vi "Setup UI.vi"(8 "error in (no error)":errorcluster, 10 "Set UI to input? (F)":bool, 11 "Wavelength in":refnum<class "Wavelength.lvclass">) -> (0 "error out":errorcluster, 3 "Wavelength out":refnum<class "Wavelength.lvclass">)   [LabVIEW 2012, in "Wavelength.lvclass"]
uses:
  Wavelength.lvclass
  Wavelength.lvclass/Wavelength.ctl
  Instruments/Spectrometer/Spectrometer Triax 550.lvclass
  Instruments/Spectrometer/JY-SPEX-TRIAX/JY-SPEX-TRIAX.lvlib
panel:
  in  "Set mirror (lateral)":bool
  in  "Go to first point":bool
  in  "Optimize":enum32{"Slits", "Step Size"}(radio)=enum."Step Size"
  out "Step size":dbl[unit] caption="Recommended step size\n(must enter above too)"
  in  "Lateral Exit":dbl[unit]
  in  "Axial Entrance":dbl[unit]
  # "Wavelength Scan Setup"
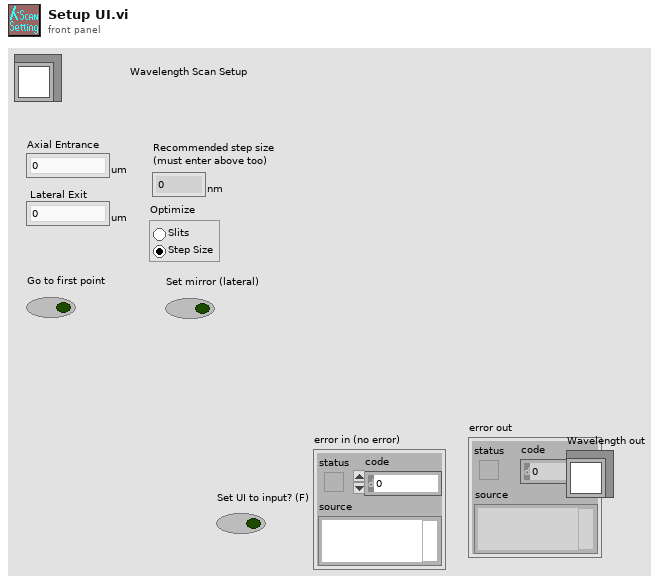
[diagram p1: front panel]
types:
  T1 = enum8{"Enabled", "Disabled", "Disabled and Grayed Out"}
  T2 = typedef "Scanner.lvclass/Range.ctl" = cluster{"xi":dbl, "xf":dbl, "dx":dbl, "Return to...?":bool, "Return to":dbl}
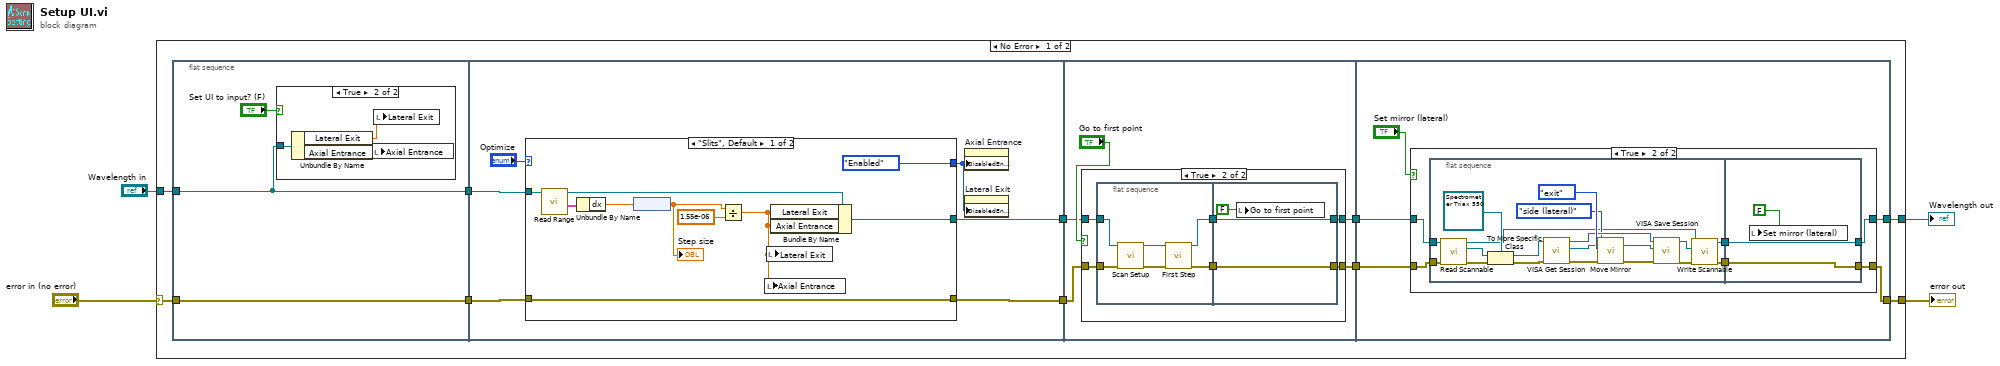
[diagram p0: block diagram]
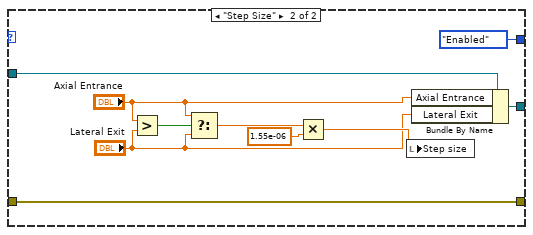
[diagram p3: hidden frame]
diagram:
  n1 = case shown="No Error" "error in (no error)" {
    selector: "error in (no error)" -> [w13 w104]
    tunnel: [w14 w104] -> w3
    tunnel: "Wavelength in" -> [w12 w105]
    tunnel: [w11 w105] -> w1
    frame No Error {
      n2 = flat-sequence {
        tunnel: w12 -> [w15]
        tunnel: w13 -> [w17]
        tunnel: [w17] -> w10
        tunnel: [w15] -> w9
        tunnel: w10 -> [w24]
        tunnel: w9 -> [w23]
        tunnel: [w25] -> w8
        tunnel: [w22] -> w7
        tunnel: w8 -> [w49]
        tunnel: w7 -> [w50]
        tunnel: [w48] -> w6
        tunnel: [w47] -> w5
        tunnel: [w73] -> w11
        tunnel: [w70] -> w14
        tunnel: w6 -> [w72]
        tunnel: w5 -> [w71]
        frame #0 {
          n3 = case shown="True" "Set UI to input? (F)" {
            tunnel: w15 -> [_ w20]
            frame False {
            }
            frame True {
              n4 = Unbundle By Name(w20) -> ("Lateral Exit"=w19:dbl[unit], "Axial Entrance"=w18:dbl[unit])
              n5 = local write "Axial Entrance"(w18) -> ()
              n6 = local write "Lateral Exit"(w19) -> ()
            }
          }
        }
        frame #1 {
          n7 = case shown="\"Slits\", Default" "Optimize" {
            tunnel: [w35 w42] -> w25
            tunnel: w24 -> [w35 w42]
            tunnel: w23 -> [w34 w43]
            tunnel: [w33 w40] -> w22
            tunnel: [T1."Enabled" ("Disabled") T1."Enabled" ("Disabled")] -> w21
            frame "Slits", Default {
              n8 = call-dynamic "Read Range.vi"("Scanner.lvclass in"=w34) -> ("Range"=w30:T2, "Scanner.lvclass out"=w31:refnum<class "Wavelength.lvclass">)  [unwired: 5 in, 4 out]
              n9 = Unbundle By Name(w30) -> ("dx"=w29:dbl)
              n10 = node(w29) -> (w28:dbl[unit])
              "Step size" <- w28
              n11 = Divide(x=w28, y=1.55e-06) -> (x/y=w32:dbl[unit])
              n12 = local write "Axial Entrance"(w32) -> ()
              n13 = local write "Lateral Exit"(w32) -> ()
              n14 = Bundle By Name(cluster=w31, "Lateral Exit"=w32, "Axial Entrance"=w32) -> (w33:refnum<class "Wavelength.lvclass">)
            }
            frame "Step Size" {
              n15 = Greater?(x="Axial Entrance", y="Lateral Exit") -> (0:w45:bool)
              n16 = Select(t="Axial Entrance", s=w45, f="Lateral Exit") -> (s? t:f=w44:dbl[unit])
              n17 = Multiply(x=w44, y=1.55e-06) -> (x*y=w41:dbl[unit])
              n18 = local write "Step size"(w41) -> ()
              n19 = Bundle By Name(cluster=w43, "Axial Entrance"="Axial Entrance", "Lateral Exit"="Lateral Exit") -> (w40:refnum<class "Wavelength.lvclass">)
            }
          }
          n20 = property on="Axial Entrance" class="DigNum (strict)"("DisabledEnum"=w21) -> ()  [unwired: 2 in, 2 out]
          n21 = property on="Lateral Exit" class="DigNum (strict)"("DisabledEnum"=w21) -> ()  [unwired: 2 in, 2 out]
        }
        frame #2 {
          n22 = case shown="True" "Go to first point" {
            tunnel: w50 -> [w53 w59]
            tunnel: w49 -> [w52 w58]
            tunnel: [w52 w57] -> w47
            tunnel: [w53 w56] -> w48
            frame False {
            }
            frame True {
              n23 = flat-sequence {
                tunnel: w59 -> [w61]
                tunnel: w58 -> [w65]
                tunnel: [w62] -> w55
                tunnel: [w60] -> w54
                tunnel: [w67] -> w56
                tunnel: [w68] -> w57
                tunnel: w55 -> [w68]
                tunnel: w54 -> [w67]
                frame #0 {
                  n24 = call-dynamic "Scan Setup.vi"("error in (no error)"=w65, "Wavelength in"=w61) -> ("error out"=w64:errorcluster, "Wavelength out"=w63:refnum<class "Wavelength.lvclass">)  [unwired: 8 in]
                  n25 = call-dynamic "First Step.vi"("error in (no error)"=w64, "Wavelength.lvclass in"=w63) -> ("error out"=w62:errorcluster, "Wavelength.lvclass out"=w60:refnum<class "Wavelength.lvclass">)  [unwired: 7 in, 1 out]
                }
                frame #1 {
                  n26 = local write "Go to first point"(FALSE ("Go to first point")) -> ()
                }
              }
            }
          }
        }
        frame #3 {
          n27 = case shown="True" "Set mirror (lateral)" {
            tunnel: [w75 w79] -> w73
            tunnel: w72 -> [w75 w81]
            tunnel: w71 -> [w74 w80]
            tunnel: [w74 w77] -> w70
            frame False {
            }
            frame True {
              n28 = flat-sequence {
                tunnel: w80 -> [w93]
                tunnel: w81 -> [w92]
                tunnel: [w83] -> w78
                tunnel: [w82] -> w76
                tunnel: [w102] -> w79
                tunnel: w78 -> [w102]
                tunnel: [w101] -> w77
                tunnel: w76 -> [w101]
                frame #0 {
                  n29 = call-dynamic "Read Scannable.vi"("error in (no error)"=w93, "Scanner.lvclass in"=w92) -> ("error out"=w91:errorcluster, "Scannable.lvclass"=w90:refnum<class "Scannable.lvclass">, "Scanner.lvclass out"=w84:refnum<class "Wavelength.lvclass">)  [unwired: 7 out]
                  n30 = To More Specific Class(target class=refnum<class "Spectrometer Triax 550.lvclass"> refnum ("Spectrometer Triax 550.lvclass"), reference=w90, error in=w91) -> (specific class reference=w87:refnum<class "Spectrometer Triax 550.lvclass">, error out=w88:errorcluster)
                  n31 = call-dynamic "VISA Get Session.vi"("error in (no error)"=w88, "Instrument.lvclass in"=w87) -> ("error out"=w98:errorcluster, "VISA Resource Name"=w99:refnum<visa-resource-name>, "Instrument.lvclass out"=w97:refnum<class "Spectrometer Triax 550.lvclass">)  [unwired: 7 out]
                  n32 = call "Move Mirror.vi"("error in (no error)"=w98, "position (side/lateral)"=enum16{"side (lateral)", "front (axial)"}."side (lateral)", "mirror (exit)"=enum16{"entrance", "exit"}."exit", "VISA resource name"=w99) -> ("error out"=w96:errorcluster, "VISA resource name out"=w95:refnum<visa-resource-name>)  [unwired: 1 in, 5 out]
                  n33 = call-dynamic "VISA Save Session.vi"("error in (no error)"=w96, "VISA Resource Name"=w95, "Instrument.lvclass in"=w97) -> ("error out"=w86:errorcluster, "Instrument.lvclass out"=w85:refnum<class "Spectrometer Triax 550.lvclass">)  [unwired: 7 out]
                  n34 = call-dynamic "Write Scannable.vi"("error in (no error)"=w86, "Scannable.lvclass"=w85, "Scanner.lvclass in"=w84) -> ("error out"=w82:errorcluster, "Scanner.lvclass out"=w83:refnum<class "Wavelength.lvclass">)  [unwired: 7 out]
                }
                frame #1 {
                  n35 = local write "Set mirror (lateral)"(FALSE ("Set mirror (laterally)")) -> ()
                }
              }
            }
          }
        }
      }
    }
    frame Error {
    }
  }
  "error out" <- w3
  "Wavelength out" <- w1
